vi "Get Joystick.vi"(8 "error in (no error)":errorcluster, 11 "XboxController-V in":refnum<class "XboxController-V.lvclass">) -> (0 "error out":errorcluster, 3 "XboxController-V out":refnum<class "XboxController-V.lvclass">)   [LabVIEW 2013, in "XboxController-V.lvclass"]
uses:
  XboxController-V.lvclass
  Logical Systems/XBoxController/XBoxController.lvclass
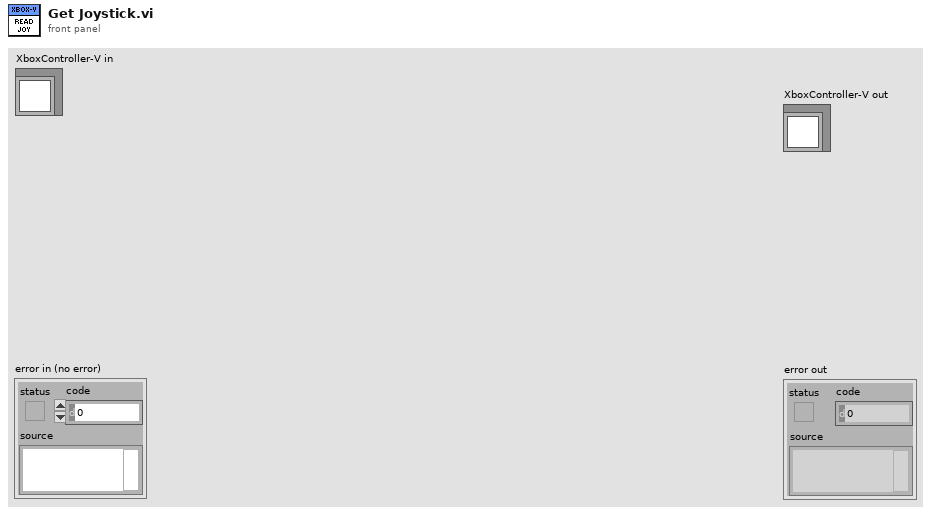
[diagram p1: front panel]
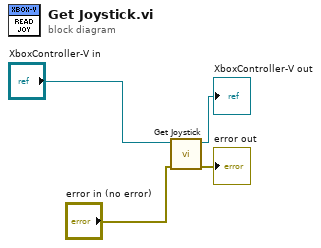
[diagram p0: block diagram]
diagram:
  n1 = call-parent "Get Joystick.vi"("error in (no error)"="error in (no error)", "XBoxController in"="XboxController-V in") -> ("error out"=→"error out":errorcluster, "XBoxController out"=→"XboxController-V out":refnum<class "XboxController-V.lvclass">)  [unwired: 8 in]
